vi "GetComand Array.vi"(8 "error in (no error)":errorcluster, 11 "reference in":refnum<class "Panel.lvclass">) -> (0 "error out":errorcluster, 2 "Comand Array":refnum<class "Command.lvclass">[](array[class]), 3 "reference out":refnum<class "Panel.lvclass">)   [LabVIEW 2013, in "Panel.lvclass"]
uses:
  Panel.lvclass
  Command_class/Command.lvclass
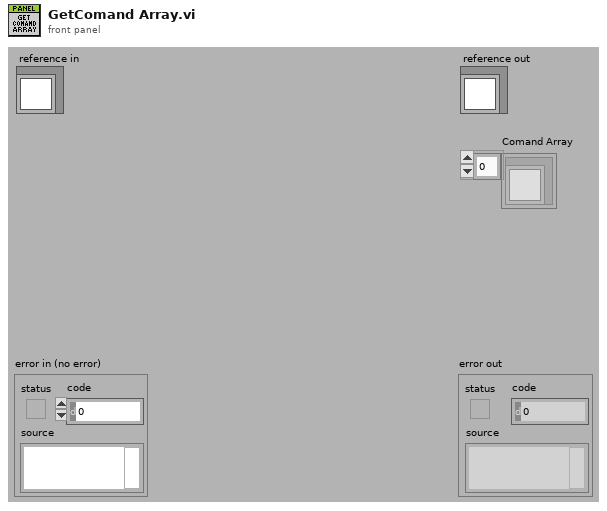
[diagram p1: front panel]
types:
  T1 = typedef "Panel.lvclass/ObjectAttributesRef.ctl" = refnum<data-value>
  T2 = typedef "Panel.lvclass/ObjectAttributes.ctl" = cluster{"Command.lvclass":refnum<class "Command.lvclass">}
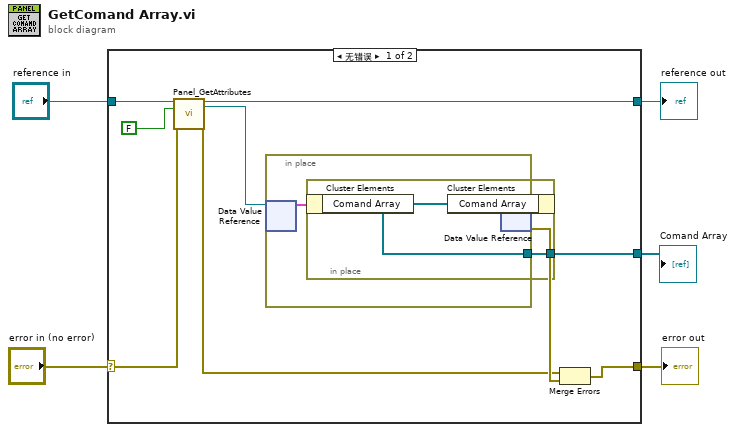
[diagram p0: block diagram]
diagram:
  n1 = case shown="无错误" "error in (no error)" {
    selector: "error in (no error)" -> [w14 w20]
    tunnel: [w8 w20] -> w4
    tunnel: [w13 w19] -> w2
    tunnel: "reference in" -> [w12 w19]
    tunnel: [w6 _] -> w1
    frame No Error {
      n2 = call "Panel_GetAttributes.vi"("reference in"=w12, "return data? (T)"=FALSE, "error in (no error)"=w14) -> ("reference out"=w13:refnum<class "Panel.lvclass">, "attributes ref"=w7:T1, "error out"=w9:errorcluster)  [unwired: 13 in, 1 out]
      n3 = in-place {
        in-place-border: [w15] -> w6
        n4 = in-place-dvr #1(w7) -> (w16:T2)  [unwired: 1 out]
        n5 = in-place {
          in-place-border: [w18] -> w15
          n6 = in-place-cluster #2(w16) -> ("Comand Array"=w18:refnum<class "Command.lvclass">[])
          n7 = in-place-cluster #2("Comand Array"=w18) -> (w17:T2)
        }
        n8 = in-place-dvr #1(w17) -> (w10:errorcluster)  [unwired: 1 out]
      }
      n9 = Merge Errors(w9, w10) -> (w8:errorcluster)
    }
    frame Error {
    }
  }
  "error out" <- w4
  "reference out" <- w2
  "Comand Array" <- w1
